vi "Host Key Fingerprint.vi"(7 "Type":T1=enum."SHA1", 8 "Error In":errorcluster, 11 "Session In":refnum<class "Session.lvclass">) -> (0 "Error Out":errorcluster, 2 "Fingerprint":u8[](array[numeric]) format="%.0x", 3 "Sesssion Out":refnum<class "Session.lvclass">)   [LabVIEW 2017, in "LabSSH2.lvlib" / "Session.lvclass"]
uses:
  Session.lvclass
  Typedefs/Host Key Hash Types.ctl
  Session.lvclass/Session.ctl
  <vilib>/Utility/error.llb/Error Cluster From Error Code.vi
  <vilib>/ErrorRing/Error Ring.xnode
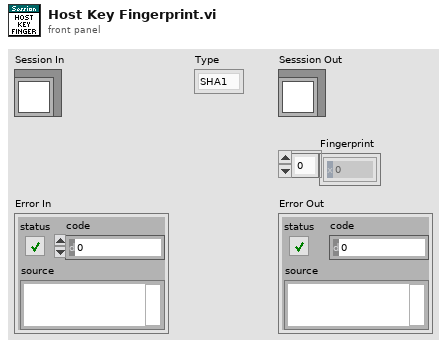
[diagram p1: front panel]
types:
  T1 = typedef "LabSSH2.lvlib/Session.lvclass/Host Key Hash Types.ctl" = enum16{"MD5", "SHA1"}
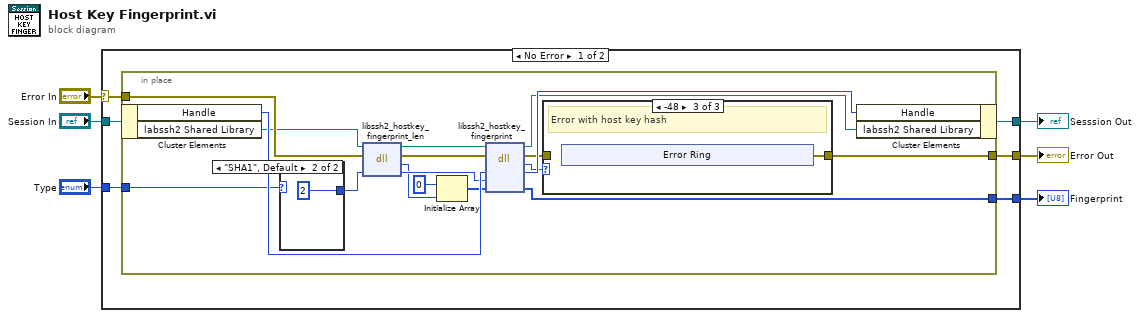
[diagram p0: block diagram]
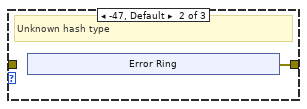
[diagram p3: hidden frame]
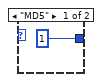
[diagram p4: hidden frame]
diagram:
  n1 = case shown="No Error" "Error In" {
    selector: "Error In" -> [w11 w44]
    tunnel: [w12 w44] -> w5
    tunnel: "Session In" -> [w10 w43]
    tunnel: [w9 w43] -> w3
    tunnel: "Type" -> [w8 _]
    tunnel: [w7 _] -> w1
    frame No Error {
      n2 = in-place {
        in-place-border: [w24] -> w12
        in-place-border: w11 -> [w22]
        in-place-border: w8 -> [w26]
        in-place-border: [w13] -> w7
        n3 = in-place-cluster #1(w10) -> ("Handle"=w29:u64, "labssh2 Shared Library"=w19:path)
        n4 = case shown="\"SHA1\", Default" w26 {
          tunnel: [1 2] -> w18
          frame "MD5" {
          }
          frame "SHA1", Default {
          }
        }
        n5 = dll-call lib="D:/Users/cfield/Code/Field R&D Services/SSH/LabSSH2/LabVIEW/trunk/src/LabSSH2/Private/labssh2.*" fn="libssh2_hostkey_fingerprint_len"(path in=w19, error in=w22, "hash_type"=w18) -> (path out=w20:path, error out=w21:errorcluster, "len"=w15:u64, "hash_type"=w17:i32)  [unwired: 1 in]
        n6 = Initialize Array(u8 0, w15) -> (w14:u8[])
        n7 = dll-call lib="D:/Users/cfield/Code/Field R&D Services/SSH/LabSSH2/LabVIEW/trunk/src/LabSSH2/Private/labssh2.*" fn="libssh2_hostkey_fingerprint"(path in=w20, error in=w21, "session"=w29, "hash_type"=w17, "buffer"=w14) -> (path out=w27:path, error out=w25:errorcluster, "result"=w23:i32, "session"=w28:u64, "buffer"=w13:u8[])  [unwired: 2 in]
        n8 = case shown="-48" w23 {
          tunnel: w25 -> [w30 _ _]
          tunnel: [w30 w31 w36] -> w24
          frame 0 {
            # "Fingerprint available, success"
          }
          frame -47, Default {
            # "Unknown hash type"
            n9 = xnode "Error Ring"() -> ("error out"=w31:errorcluster)
          }
          frame -48 {
            # "Error with host key hash"
            n10 = xnode "Error Ring"() -> ("error out"=w36:errorcluster)
          }
        }
        n11 = in-place-cluster #1("Handle"=w28, "labssh2 Shared Library"=w27) -> (w9:refnum<class "Session.lvclass">)
      }
    }
    frame Error {
    }
  }
  "Sesssion Out" <- w3
  "Error Out" <- w5
  "Fingerprint" <- w1
